vi "Data_Acquisition.vi"(11 "Error_In":errorcluster) -> (15 "Error_Out":errorcluster)   [LabVIEW 2023]
doc: "This VI Generate or simulate the data and transfer to MainVI."
uses:
  Controls/Main_Status.ctl
  Controls/Generated_data.ctl
  Controls/Queue_Operation.ctl
  <vilib>/numeric/Random Number (Range) DBL.vi
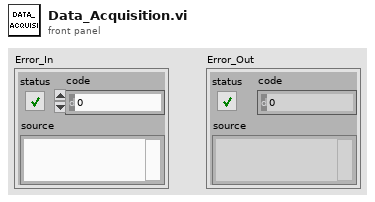
[diagram p1: front panel]
types:
  T1 = typedef "Main_Status.ctl" = cluster{"Stop?":bool, "Start/Stop_Acquisition ":bool, "Wait_Time":i32}
  T2 = typedef "Generated_data.ctl" = cluster{"Current_Data":dbl, "Temp_Data":dbl}
  T3 = typedef "Queue_Operation.ctl" = enum16{"Obtain_Queue", "Enqueue", "Lossy_Enqueue", "Preview", "Queue_Status", "Release_Queue", "Dequeue", "Flush"}
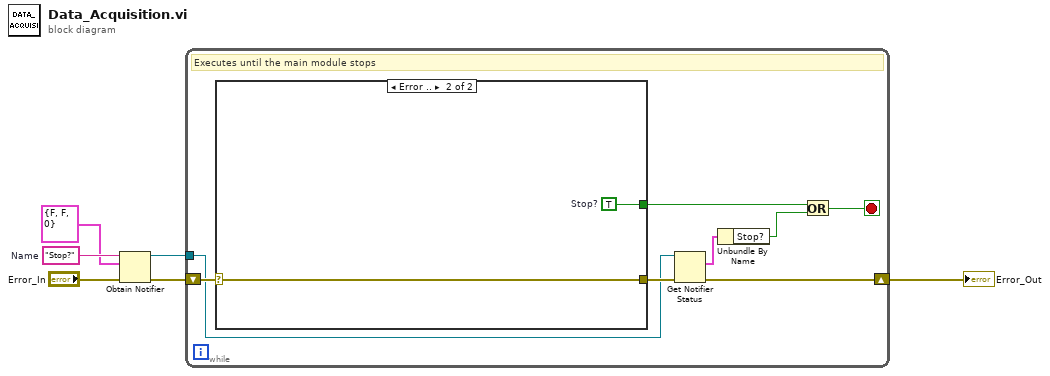
[diagram p0: block diagram]
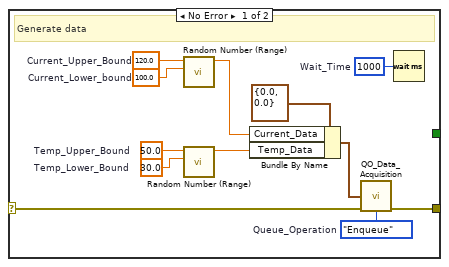
[diagram p2: hidden frame]
diagram:
  w3 = "Stop?"  # Name
  n1 = Obtain Notifier(name (unnamed)=w3, notification data type=T1 {"Stop?"=FALSE, "Start/Stop_Acquisition "=FALSE, "Wait_Time"=0} ("Cluster"), error in (no error)="Error_In") -> (notifier out=w4:refnum<notifier>, error out=w5:errorcluster)  [unwired: 1 in, 1 out]
  n2 = while {
    tunnel: w4 -> [w11]
    shift-right: [w12] -> w1
    shift-left: w5 -> [w14]
    stop <- w7 stop-if-true
    # "Executes until the main module stops"
    n3 = case shown="Error .." w14 {
      selector: w14 -> [w16 w28]
      tunnel: [w15 w28] -> w13
      tunnel: [_ w27] -> w9
      frame No Error {
        w17 = u32 1000  # Wait_Time
        w19 = Queue_Operation."Enqueue"  # Queue_Operation
        w23 = 30.0  # Temp_Lower_Bound
        w24 = 50.0  # Temp_Upper_Bound
        w25 = 100.0  # Current_Lower_bound
        w26 = 120.0  # Current_Upper_Bound
        # "Generate data"
        n4 = call-poly <vilib>:"Random Number (Range).vi"("lower bound (0)"=w25, "upper bound (100)"=w26) -> ("number"=w22:dbl)  [unwired: 9 in]
        n5 = call-poly <vilib>:"Random Number (Range).vi"("lower bound (0)"=w23, "upper bound (100)"=w24) -> ("number"=w21:dbl)  [unwired: 9 in]
        n6 = Bundle By Name(cluster=T2 {"Current_Data"=0.0, "Temp_Data"=0.0} ("Generated_Data"), "Current_Data"=w22, "Temp_Data"=w21) -> (w18:T2)
        n7 = call "QO_Data_Acquisition.vi"("Data_In"=w18, "Error_In"=w16, "Queue_Operation"=w19) -> ("Error_Out"=w15:errorcluster)  [unwired: 8 in, 4 out]
        n8 = Wait (ms)(milliseconds to wait=w17) -> ()  [unwired: 1 out]
      }
      frame Error {
        w27 = TRUE  # Stop?
      }
    }
    n9 = Get Notifier Status(notifier=w11, error in (no error)=w13) -> (current notification=w10:T1, error out=w12:errorcluster)  [unwired: 3 out]
    n10 = Unbundle By Name(w10) -> ("Stop?"=w8:bool)
    n11 = Or(x=w9, y=w8) -> (x .or. y?=w7:bool)
  }
  "Error_Out" <- w1
